vi "LCP Enable Force Monitoring.vi"(7 "Enable":bool, 8 "error in (no error)":errorcluster caption="Fehler (Eingang, kein Fehler)", 11 "Pump Handle":i64) -> (0 "error out":errorcluster caption="Fehler (Ausgang)")   [LabVIEW 2021, in "labbCAN_Pump_API.lvlib"]
doc: "LCP_Func long LCP_CALL LCP_Enable(dev_hdl hPump);"
uses:
  labbCAN_Pump_API.lvlib
  labbCAN_Pump_API.dll
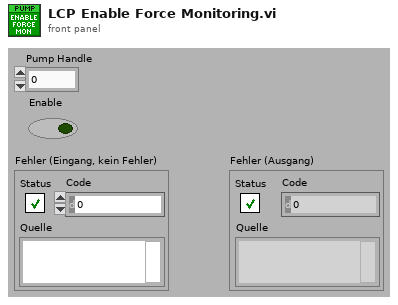
[diagram p1: front panel]
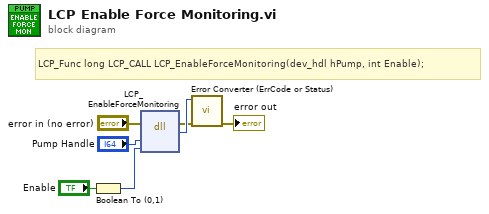
[diagram p0: block diagram]
diagram:
  # "LCP_Func long LCP_CALL LCP_EnableForceMonitoring(dev_hdl hPump, int Enable);"
  n1 = Boolean To (0,1)(Boolean="Enable") -> (0, 1=w1:i16)
  n2 = dll-call lib="C:/Users/olaja/AppData/Local/CETONI_SDK/labbCAN_Pump_API.*" fn="LCP_EnableForceMonitoring"(error in="error in (no error)", "hPump"="Pump Handle", "Enable"=w1) -> (error out=w4:errorcluster, "Rückgabetyp"=w5:i32)  [unwired: 4 in, 1 out]
  n3 = call "Error Converter (ErrCode or Status).vi"("error in (no error)"=w4, "error code"=w5) -> ("error out"=→"error out":errorcluster)  [unwired: 9 in]
